vi "ziModExecute.vi"(7 "Error In":errorcluster, 9 "Modal (F)":bool, 10 "ziModHandle In":T1 {"ModHandle" format="0x%08x"; "Conn" format="0x%08x"}) -> (0 "Error Out":errorcluster, 2 "Finished?":bool, 3 "ziModHandle Out":T1 {"ModHandle" format="0x%08x"; "Conn" format="0x%08x"})   [LabVIEW 2015, in "Zurich Instruments LabOne.lvlib"]
doc: "Start the module. If the <b>Modal</b> is set to false, the vi waits for the module to finish and polls the data from the device. Use ziModGetNextNode.vi in order to access the availible data. If the <b>Modal</b> is set to true, the module is started. In order to poll the data from the device use ziModRead.vi."
uses:
  Zurich Instruments LabOne.lvlib
  Zurich Instruments/LabOne/API/LabVIEW/Zurich Instruments LabOne/Private/ziLV64.framework
  ziTypeModHandle.ctl
panel:
  in  "stop":bool
  out "Progress (unity)":dbl
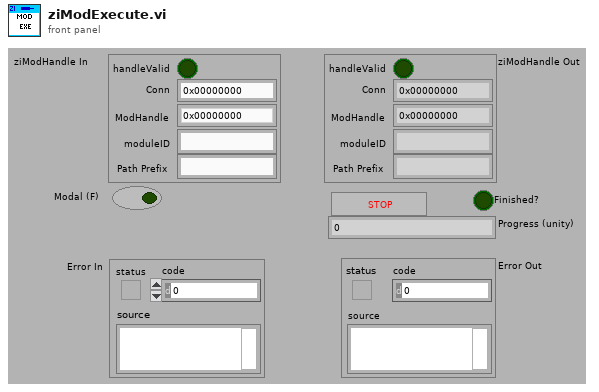
[diagram p1: front panel]
types:
  T1 = typedef "Zurich Instruments LabOne.lvlib/ziTypeModHandle.ctl" = cluster{"handleValid":bool, "Conn":u64, "ModHandle":u64, "moduleID":string, "Path Prefix":string}
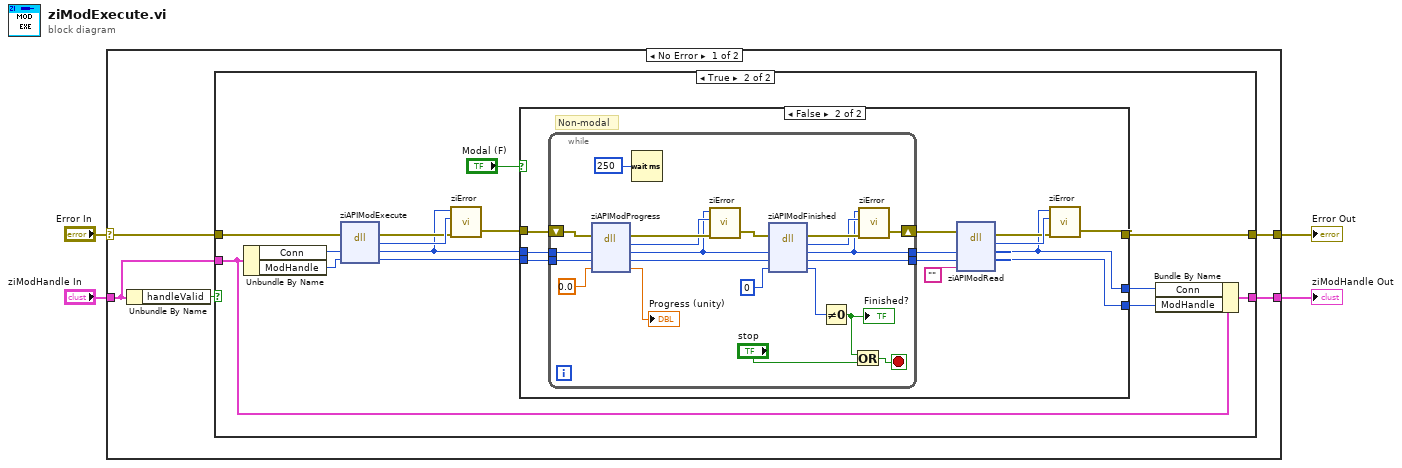
[diagram p0: block diagram]
diagram:
  n1 = case shown="No Error" "Error In" {
    selector: "Error In" -> [w7 w63]
    tunnel: "ziModHandle In" -> [w6 w62]
    tunnel: [w9 w62] -> w1
    tunnel: [w8 w63] -> w4
    frame No Error {
      n2 = Unbundle By Name(w6) -> ("handleValid"=w5:bool)
      n3 = case shown="True" w5 {
        tunnel: w6 -> [w11 w22]
        tunnel: [w11 w21] -> w9
        tunnel: w7 -> [w10 w25]
        tunnel: [w10 w13] -> w8
        frame False {
        }
        frame True {
          n4 = Unbundle By Name(w22) -> ("Conn"=w24:u64, "ModHandle"=w23:u64)
          n5 = dll-call lib="Users/arkady/Desktop/ado/github/resonant_ultrasound_arxiv/maglab ultrasound -- arkady --arxiv/Zurich Instruments/LabOne/API/LabVIEW/Zurich Instruments LabOne/Private/ziLV*.*" fn="ziAPIModExecute"(error in=w25, "conn"=w24, "ModHandle"=w23) -> (error out=w15:errorcluster, "return type"=w16:u32, "conn"=w12:u64, "ModHandle"=w20:u64)  [unwired: 2 in, 1 out]
          n6 = call "ziError.vi"("Conn"=w12, "ziErrorCode"=w16, "Error In"=w15) -> ("Error Out"=w14:errorcluster)  [unwired: 2 in, 1 out]
          n7 = case shown="False" "Modal (F)" {
            tunnel: w12 -> [w27 w40]
            tunnel: w20 -> [w26 w39]
            tunnel: [w28 w30] -> w13
            tunnel: [w26 w34] -> w19
            tunnel: [w27 w29] -> w18
            tunnel: w14 -> [w28 w33]
            frame True {
            }
            frame False {
              # "Non-modal"
              n8 = while {
                tunnel: w40 -> [w60]
                tunnel: w39 -> [w59]
                tunnel: [w61] -> w35
                tunnel: [w41] -> w36
                shift-right: [w46] -> w37
                shift-left: w33 -> [w49]
                stop <- w44 stop-if-true
                n9 = dll-call lib="Users/arkady/Desktop/ado/github/resonant_ultrasound_arxiv/maglab ultrasound -- arkady --arxiv/Zurich Instruments/LabOne/API/LabVIEW/Zurich Instruments LabOne/Private/ziLV*.*" fn="ziAPIModProgress"(error in=w49, "conn"=w60, "ModHandle"=w59, "Finished"=0.0) -> (error out=w55:errorcluster, "return type"=w53:u32, "conn"=w42:u64, "ModHandle"=w58:u64, "Finished"=→"Progress (unity)":dbl)  [unwired: 2 in, 1 out]
                n10 = Wait (ms)(milliseconds to wait=u32 250) -> ()  [unwired: 1 out]
                n11 = call "ziError.vi"("Conn"=w42, "ziErrorCode"=w53, "Error In"=w55) -> ("Error Out"=w54:errorcluster)  [unwired: 2 in, 1 out]
                n12 = dll-call lib="Users/arkady/Desktop/ado/github/resonant_ultrasound_arxiv/maglab ultrasound -- arkady --arxiv/Zurich Instruments/LabOne/API/LabVIEW/Zurich Instruments LabOne/Private/ziLV*.*" fn="ziAPIModFinished"(error in=w54, "conn"=w42, "ModHandle"=w58, "Finished"=i64 0) -> (error out=w52:errorcluster, "return type"=w51:u32, "conn"=w41:u64, "ModHandle"=w61:u64, "Finished"=w56:i64)  [unwired: 2 in, 1 out]
                n13 = Not Equal To 0?(x=w56) -> (x != 0?=w45:bool)
                "Finished?" <- w45
                n14 = Or(x=w45, y="stop") -> (x .or. y?=w44:bool)
                n15 = call "ziError.vi"("Conn"=w41, "ziErrorCode"=w51, "Error In"=w52) -> ("Error Out"=w46:errorcluster)  [unwired: 2 in, 1 out]
              }
              n16 = dll-call lib="Users/arkady/Desktop/ado/github/resonant_ultrasound_arxiv/maglab ultrasound -- arkady --arxiv/Zurich Instruments/LabOne/API/LabVIEW/Zurich Instruments LabOne/Private/ziLV*.*" fn="ziAPIModRead"(error in=w37, "Conn"=w36, "ModHandle"=w35, "Path"="") -> (error out=w31:errorcluster, "return type"=w32:u32, "Conn"=w29:u64, "ModHandle"=w34:u64)  [unwired: 3 in, 1 out]
              n17 = call "ziError.vi"("Conn"=w29, "ziErrorCode"=w32, "Error In"=w31) -> ("Error Out"=w30:errorcluster)  [unwired: 2 in, 1 out]
            }
          }
          n18 = Bundle By Name(cluster=w22, "Conn"=w18, "ModHandle"=w19) -> (w21:T1)
        }
      }
    }
    frame Error {
    }
  }
  "Error Out" <- w4
  "ziModHandle Out" <- w1
